vi "Register Process.vi"(6 "Forces Self to Run (F)":bool, 7 "Parent Call":T1, 8 "error in (no error)":errorcluster, 9 "Process Name (optional)":string, 11 "SMO":refnum<class "SMO.lvclass">) -> (0 "error out":errorcluster, 3 "SMO out":refnum<class "SMO.lvclass">)   [LabVIEW 2021, in "smo.lvlib" / "SMO.lvclass"]
doc: "Philosophy of Registration of SMOs\n=========================\nOverriding \"Process.vi\" is mandatory (Must Call Parent) to allow the framework to achieve necessary housekeeping functionality.\nThere are two ways the developer can override a process: a) by extending its functionalities (EXTENSION) or b) by overwriting its functionalities (OVERWRITE).\nEven if the parent method has to be called, the framework allows the developer to request that its parent process not run (overwriting).\n\nAt this point, it becomes the responsibility of the parent process to decide if it should comply with this request or ignore it. If it chooses to ignore its child's request,\nthe process will be extended. This is meant to allow a process to do critical functions necessary to its performance even if the child requests to overwrite it.\n\nIn a nutshell, each process can decide at runtime if it allows itself to be overwritten or simply extended by a more specific implementation."
uses:
  SMO.lvclass
  Typedefs/Parent Call--Enum.ctl
  SMO.lvclass/SMO.ctl
  Private/ReftoDVR--SMO.vi
  <vilib>/Utility/error.llb/Clear Errors.vi
panel:
  # "For instructions on how to use the JKI State Machine Objects, examples and video tutorials, visit:\nhttp://jki.net/state-machine-objects/\n\nJKI State Machine Objects™\nhttp://jki.net/state-machine-objects/\nCopyright (C) 2005-2015, JKI <info@jki.net>\nALL RIGHTS RESERVED"
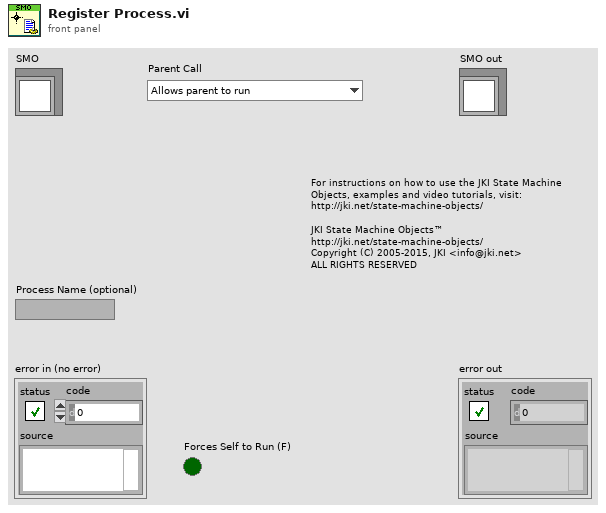
[diagram p1: front panel]
types:
  T1 = typedef "smo.lvlib/SMO.lvclass/Parent Call--Enum.ctl" = enum16{"Allows parent to run", "Does not request parent to run"}
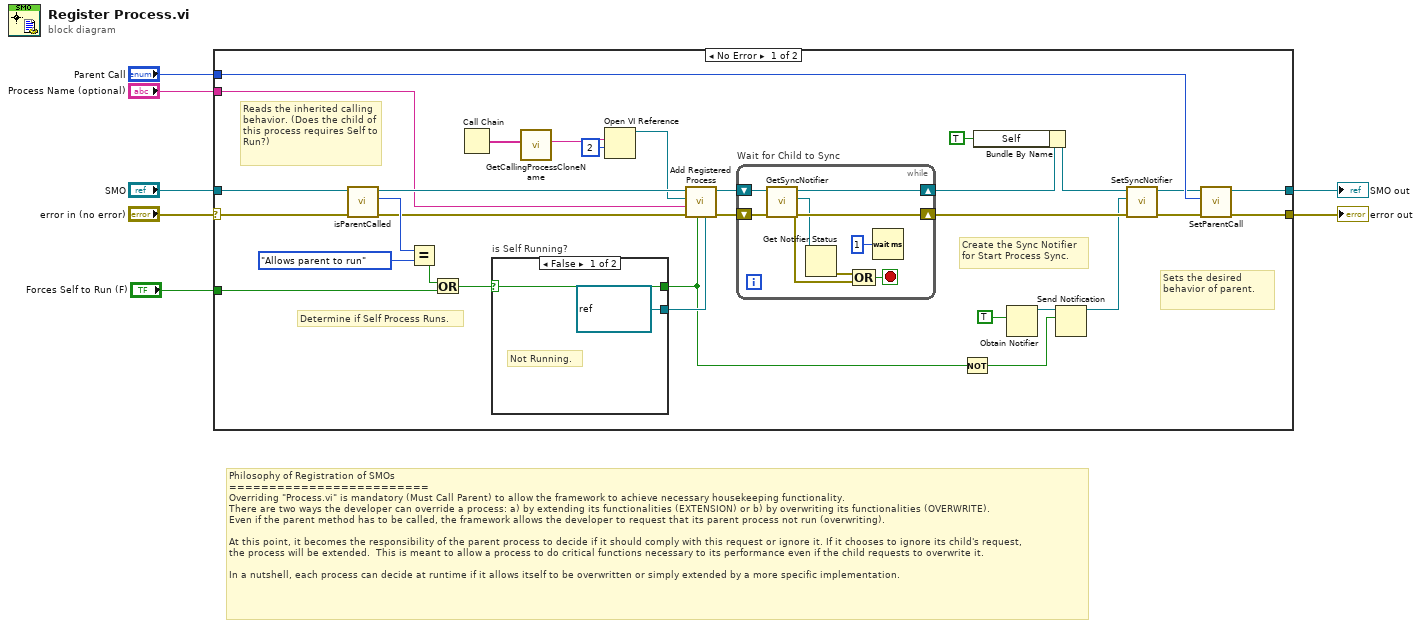
[diagram p0: block diagram]
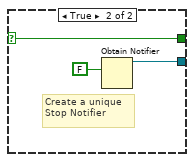
[diagram p2: hidden frame]
diagram:
  # "Philosophy of Registration of SMOs\n=========================\nOverriding \"Process.vi\" is mandatory (Must Call Parent) to allow the framework to achieve necessary housekeeping functionality.\nThere are two ways the developer can override a process: a) by extending its functionalities (EXTENSION) or b) by overwriting its functionalities (OVERWRITE).\nEven if the parent method has to be called, the framework allows the developer to request that its parent process not run (overwriting).\n\nAt this point, it becomes the responsibility of the parent process to decide if it should comply with this request or ignore it. If it chooses to ignore its child's request,\nthe process will be extended.  This is meant to allow a process to do critical functions necessary to its performance even if the child requests to overwrite it.\n\nIn a nutshell, each process can decide at runtime if it allows itself to be overwritten or simply extended by a more specific implementation."
  n1 = case shown="No Error" "error in (no error)" {
    selector: "error in (no error)" -> [w23 w52]
    tunnel: "SMO" -> [w24 w53]
    tunnel: [w31 w53] -> w6
    tunnel: [w30 w52] -> w4
    tunnel: "Process Name (optional)" -> [w25 _]
    tunnel: "Parent Call" -> [w37 _]
    tunnel: "Forces Self to Run (F)" -> [w35 _]
    frame No Error {
      # "Create the Sync Notifier\nfor Start Process Sync."
      # "Determine if Self Process Runs."
      # "Sets the desired behavior of parent."
      # "Reads the inherited calling behavior. (Does the child of this process requires Self to Run?)"
      n2 = call "isParentCalled.vi"("error in (no error)"=w23, "SMO in"=w24) -> ("error out"=w27:errorcluster, "Parent Call"=w38:T1, "SMO out"=w28:refnum<class "SMO.lvclass">)  [unwired: 7 in]
      n3 = Equal?(x=w38, y=Parent_Call--Enum."Allows parent to run") -> (x = y?=w36:bool)
      n4 = Or(x=w36, y=w35) -> (x .or. y?=w21:bool)
      n5 = Call Chain() -> (call chain=w9:string[])
      n6 = case "is Self Running?" shown="False" w21 {
        selector: w21 -> [w48 w50]
        tunnel: [refnum<notifier> refnum ("notifier out") w51] -> w22
        tunnel: [w48 w50] -> w12
        frame False {
          # "Not Running."
        }
        frame True {
          # "Create a unique Stop Notifier"
          n7 = Obtain Notifier(notification data type=FALSE) -> (notifier out=w51:refnum<notifier>)  [unwired: 3 in, 2 out]
        }
      }
      n8 = call "GetCallingProcessCloneName.vi"("call chain"=w9) -> ("Process Clone"=w8:string)  [unwired: 10 in]
      n9 = Open VI Reference(vi path=w8, options=2) -> (vi reference=w26:refnum<vi>)  [unwired: 4 in, 1 out]
      n10 = call "Add Registered Process.vi"("Sync Notifier"=w22, "Process Runs (T)"=w12, "error in (no error)"=w27, "Process Name (Optional)"=w25, "Process VI (Static VI Ref)"=w26, "SMO"=w28) -> ("error out"=w19:errorcluster, "SMO out"=w20:refnum<class "SMO.lvclass">)  [unwired: 4 in]
      n11 = while "Wait for Child to Sync" {
        shift-right: [w45] -> w16
        shift-left: w20 -> [w46]
        shift-right: [w42] -> w18
        shift-left: w19 -> [w44]
        stop <- w43 stop-if-true
        n12 = call "GetSyncNotifier.vi"("error in (no error)"=w44, "SMO in"=w46) -> ("error out"=w42:errorcluster, "Sync Notifier"=w40:refnum<notifier>, "SMO out"=w45:refnum<class "SMO.lvclass">)  [unwired: 7 in]
        n13 = Get Notifier Status(notifier=w40) -> (error out=w39:errorcluster)  [unwired: 1 in, 4 out]
        n14 = Compound Arithmetic op=OR(w39, w42) -> (w43:bool)
        n15 = Wait (ms)(milliseconds to wait=u32 1) -> ()  [unwired: 1 out]
      }
      n16 = Not(x=w12) -> (.not. x?=w11:bool)
      n17 = Bundle By Name(cluster=w16, "Self"=TRUE ("Reserved.Self")) -> (w15:refnum<class "SMO.lvclass">)
      n18 = Obtain Notifier(notification data type=TRUE) -> (notifier out=w13:refnum<notifier>)  [unwired: 3 in, 2 out]
      n19 = Send Notification(notification=w11, notifier=w13) -> (notifier out=w10:refnum<notifier>)  [unwired: 1 in, 1 out]
      n20 = call "SetSyncNotifier.vi"("error in (no error)"=w18, "Sync Notifier"=w10, "SMO in"=w15) -> ("error out"=w32:errorcluster, "SMO out"=w33:refnum<class "SMO.lvclass">)  [unwired: 7 in]
      n21 = call "SetParentCall.vi"("error in (no error)"=w32, "Parent Call"=w37, "SMO in"=w33) -> ("error out"=w30:errorcluster, "SMO out"=w31:refnum<class "SMO.lvclass">)  [unwired: 7 in]
    }
    frame Error {
    }
  }
  "error out" <- w4
  "SMO out" <- w6
